vi "execute_script.vi"(8 "error in (no error)":errorcluster, 11 "preregistraion_data":T1) -> (0 "error out":errorcluster)   [LabVIEW 2018]
uses:
  controls/preregistration_data.ctl
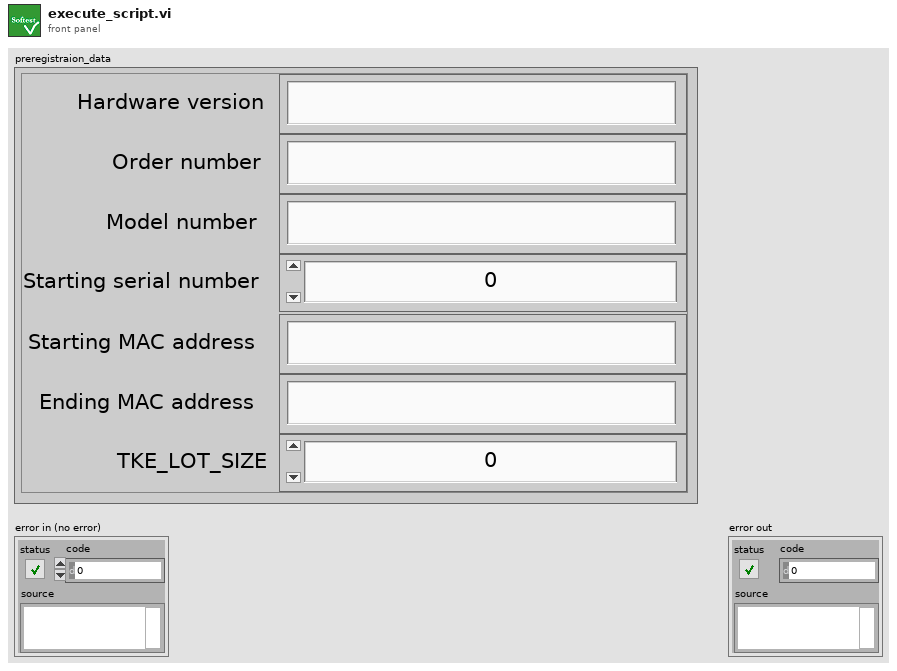
[diagram p1: front panel]
types:
  T1 = typedef "preregistration_data.ctl" = cluster{"Hardware version":string, "Order number":string, "Model number":string, "Starting serial number":i32, "Starting MAC address":string, "Ending MAC address":string, "TKE_LOT_SIZE":i32}
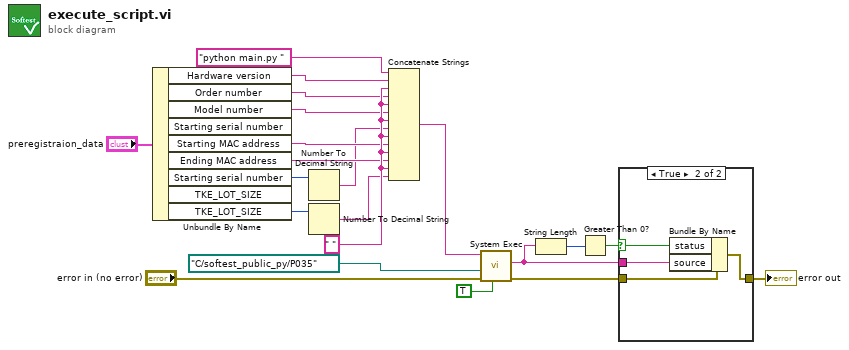
[diagram p0: block diagram]
diagram:
  w17 = " "
  n1 = Unbundle By Name("preregistraion_data") -> ("Hardware version"=w10:string, "Order number"=w11:string, "Model number"=w12:string, "Starting MAC address"=w14:string, "Ending MAC address"=w15:string, "Starting serial number"=w19:i32, "TKE_LOT_SIZE"=w20:i32)  [unwired: 2 out]
  n2 = Number To Decimal String(number=w19) -> (decimal integer string=w13:string)  [unwired: 1 in]
  n3 = Number To Decimal String(number=w20) -> (decimal integer string=w16:string)  [unwired: 1 in]
  n4 = Concatenate Strings("python main.py " ("string"), w10, w17, w11, w17, w12, w17, w13, w17, w14, w17, w15, w17, w16) -> (w18:string)
  n5 = call <vilib>:"System Exec.vi"("run minimized? (F)"=TRUE, "error in (no error)"="error in (no error)", "working directory"=path "C:/softest_public_py/P035" ("module path"), "command line"=w18) -> ("error out"=w3:errorcluster, "standard error"=w1:string)  [unwired: 4 in, 2 out]
  n6 = String Length(string=w1) -> (length=w5:i32)
  n7 = Greater Than 0?(x=w5) -> (x > 0?=w4:bool)
  n8 = case shown="True" w4 {
    selector: w4 -> [_ w23]
    tunnel: w3 -> [w22 w26]
    tunnel: [w22 w25] -> w2
    tunnel: w1 -> [_ w24]
    frame False {
    }
    frame True {
      n9 = Bundle By Name(cluster=w26, "status"=w23, "source"=w24) -> (w25:errorcluster)
    }
  }
  "error out" <- w2
